vi "Build Unconfigured Config.vi"(8 "error in (no error)":errorcluster, 11 "Volatus Core in":refnum<class "Volatus Core.lvclass">) -> (0 "error out":errorcluster, 3 "Volatus Core out":refnum<class "Volatus Core.lvclass">)   [LabVIEW 2020, in "Volatus.lvlib" / "Volatus Core.lvclass"]
uses:
  Volatus Core.lvclass
  Volatus Core.lvclass/Volatus Core.ctl
  VolatusConfig/Cluster/Cluster Config.lvclass
  VolatusConfig/VolatusConfig/VolatusConfig.lvclass
  VolatusConfig/Node/Node Config.lvclass
  lv-vecto/Vecto/Node Config/TCP Messaging Info.ctl
  lv-vecto/VectoConfig/VectoConfig.lvlib
  VolatusConfig/System/System Config.lvclass
  Module/Module.lvclass
  lv-vecto/VectoConfig/Endpoint.ctl
  C:/dev/lv20CE/relink/lv-volatus/VolatusConfig/VolatusConfigElement/VolatusConfigElement.lvclass
  C:/dev/lv20CE/relink/lv-volatus/VolatusConfig/Node/Node Config.lvclass
  C:/dev/lv20CE/relink/lv-volatus/Volatus/Module/Module.lvclass
  C:/dev/lv20CE/relink/lv-volatus/Volatus/Volatus Core/Volatus Core.lvclass
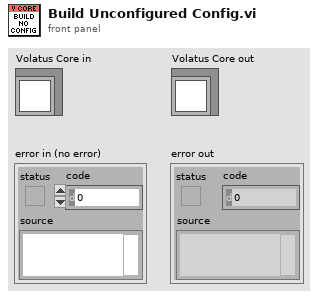
[diagram p1: front panel]
types:
  T1 = typedef "VectoConfig.lvlib/TCP Messaging Info.ctl" = cluster{"Address":string, "Port":u16, "Server (Client)":bool}
  T2 = typedef "VectoConfig.lvlib/Endpoint.ctl" = cluster{"Address":string, "Port":u16}
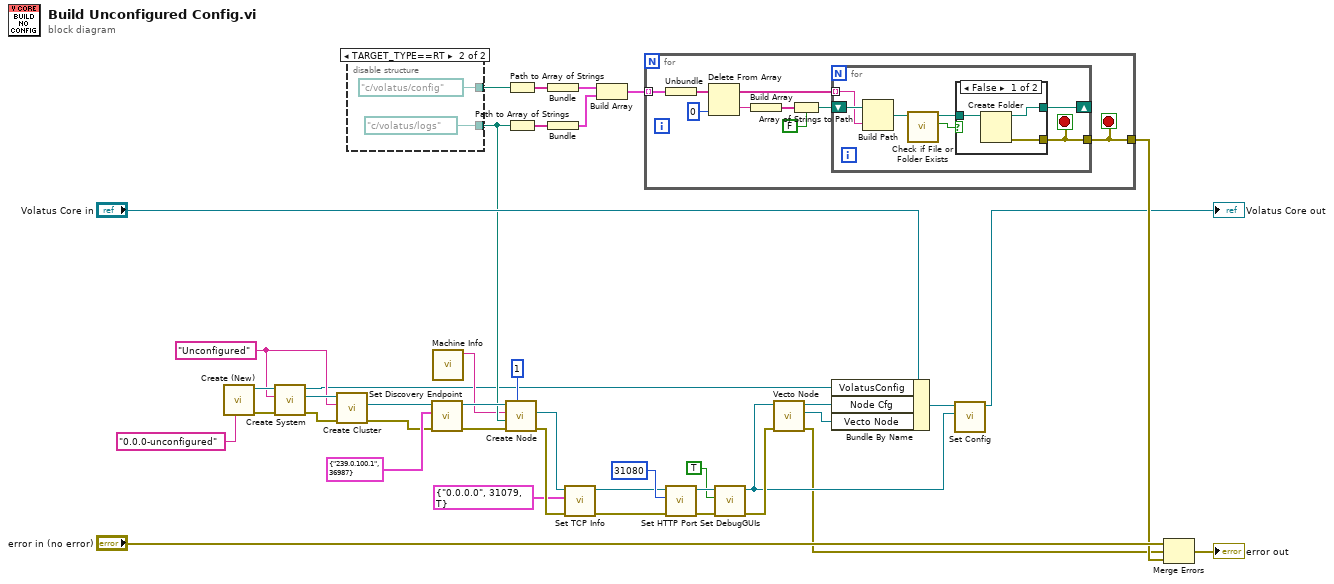
[diagram p0: block diagram]
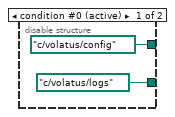
[diagram p3: hidden frame]
diagram:
  w8 = "Unconfigured"
  n1 = call "Create (New).vi"("Config Version (0.0.0)"="0.0.0-unconfigured") -> ("error out"=w35:errorcluster, "VolatusConfig out"=w36:refnum<class "VolatusConfig.lvclass">)  [unwired: 9 in]
  n2 = call "Create System.vi"("error in (no error)"=w35, "System Name"=w8, "VolatusConfig in"=w36) -> ("error out"=w20:errorcluster, "System"=w21:refnum<class "System Config.lvclass">, "VolatusConfig out"=w4:refnum<class "VolatusConfig.lvclass">)  [unwired: 6 in]
  n3 = call "Create Cluster.vi"("error in (no error)"=w20, "Cluster Name"=w8, "System in"=w21) -> ("error out"=w18:errorcluster, "Cluster"=w19:refnum<class "Cluster Config.lvclass">)  [unwired: 6 in, 1 out]
  n4 = disable-structure shown="TARGET_TYPE==RT" {
    disable-tunnel: [path "c:/volatus/config" path "c:/volatus/config"] -> w28
    disable-tunnel: [path "c:/volatus/logs" path "c:/volatus/logs"] -> w16
    frame condition #0 (active) {
    }
    frame condition #1 {
    }
  }
  n5 = call "Set Discovery Endpoint.vi"("error in (no error)"=w18, "Discovery Endpoint"=T2 {"Address"="239.0.100.1", "Port"=36987}, "Cluster in"=w19) -> ("error out"=w14:errorcluster, "Cluster out"=w17:refnum<class "Cluster Config.lvclass">)  [unwired: 7 in]
  n6 = call "Machine Info.vi"() -> ("Machine ID"=w9:string)  [unwired: 8 in, 3 out]
  n7 = call "Create Node.vi"("Node ID"=u32 1, "error in (no error)"=w14, "Event Log Folder"=w16, "Node Name"=w9, "Cluster in"=w17) -> ("error out"=w40:errorcluster, "Node"=w13:refnum<class "Node Config.lvclass">)  [unwired: 4 in, 1 out]
  n8 = Path to Array of Strings(0:w28) -> (2:w23:string[])  [unwired: 1 out]
  n9 = Path to Array of Strings(0:w16) -> (2:w24:string[])  [unwired: 1 out]
  n10 = Bundle("array of strings"=w23) -> (w27:cluster{"array of strings":string[]})  [unwired: 1 in]
  n11 = Bundle("array of strings"=w24) -> (w26:cluster{"array of strings":string[]})  [unwired: 1 in]
  n12 = call "Set TCP Info.vi"("error in (no error)"=w40, "TCP Messaging Info"=T1 {"Address"="0.0.0.0", "Port"=31079, "Server (Client)"=TRUE}, "Node in"=w13) -> ("error out"=w1:errorcluster, "Node out"=w2:refnum<class "Node Config.lvclass">)  [unwired: 7 in]
  n13 = Build Array(w27, w26) -> (w25:cluster{"array of strings":string[]}[])
  n14 = for {
    tunnel: w25 -> [w54] mode=indexing
    tunnel: [w50] -> w22
    stop <- w50 stop-if-true
    n15 = Unbundle(w54) -> ("array of strings"=w53:string[])
    n16 = Delete From Array(array=w53, index=0) -> (deleted portion=w49:string, array with subset deleted=w51:string[])  [unwired: 1 in]
    n17 = Build Array(w49) -> (w48:string[])
    n18 = Array of Strings to Path(0:w48, 1:FALSE ("relative")) -> (2:w46:path)
    n19 = for {
      shift-right: [w57] -> _
      shift-left: w46 -> [w61]
      tunnel: w51 -> [w60] mode=indexing
      tunnel: [w55] -> w50
      stop <- w55 stop-if-true
      n20 = Build Path(base path=w61, name or relative path=w60) -> (appended path=w59:path)
      n21 = call <vilib>:"Check if File or Folder Exists.vi"("path"=w59) -> ("file or folder exists?"=w58:bool, "dup path"=w56:path)  [unwired: 8 in, 1 out]
      n22 = case shown="False" w58 {
        tunnel: [w63 w65] -> w57
        tunnel: w56 -> [w64 w65]
        tunnel: [w62 _] -> w55
        frame False {
          n23 = Create Folder(path (use dialog)=w64) -> (created path=w63:path, error out=w62:errorcluster)  [unwired: 2 in, 1 out]
        }
        frame True {
        }
      }
    }
  }
  n24 = call "Set HTTP Port.vi"("error in (no error)"=w1, "HTTP Port"=u16 31080, "Node in"=w2) -> ("error out"=w32:errorcluster, "Node out"=w31:refnum<class "Node Config.lvclass">)  [unwired: 7 in]
  n25 = call "Set DebugGUIs.vi"("error in (no error)"=w32, "DebugGUIs"=TRUE, "Node in"=w31) -> ("error out"=w41:errorcluster, "Node out"=w10:refnum<class "Node Config.lvclass">)  [unwired: 7 in]
  n26 = call "Vecto Node.vi"("error in (no error)"=w41, "Node in"=w10) -> ("error out"=w3:errorcluster, "Vecto Node"=w5:refnum<class "Node Config.lvclass">, "Node out"=w6:refnum<class "Node Config.lvclass">)  [unwired: 7 in]
  n27 = Bundle By Name(cluster="Volatus Core in", "VolatusConfig"=w4, "Node Cfg"=w6, "Vecto Node"=w5) -> (w12:refnum<class "Volatus Core.lvclass">)
  n28 = call "Set Config.vi"("Config"=w10, "Module in"=w12) -> ("Module out"=→"Volatus Core out":refnum<class "Volatus Core.lvclass">)  [unwired: 9 in]
  n29 = Merge Errors("error in (no error)", w3, w22) -> (→"error out":errorcluster)
